vi "ReadUserExpressions.vi"(8 "error in (no error)":errorcluster, 11 "object in":refnum<class "execute_reply Message.lvclass">) -> (0 "error out":errorcluster, 2 "User Expressions":variant, 3 "object out":refnum<class "execute_reply Message.lvclass">)   [LabVIEW 2018, in "ClientMessaging.lvlib" / "execute_reply Message.lvclass"]
uses:
  execute_reply Message.lvclass
  execute_reply Message.lvclass/execute_reply Message.ctl
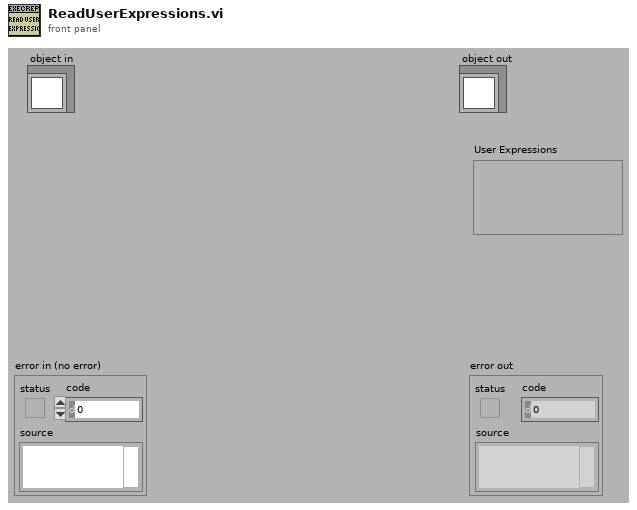
[diagram p1: front panel]
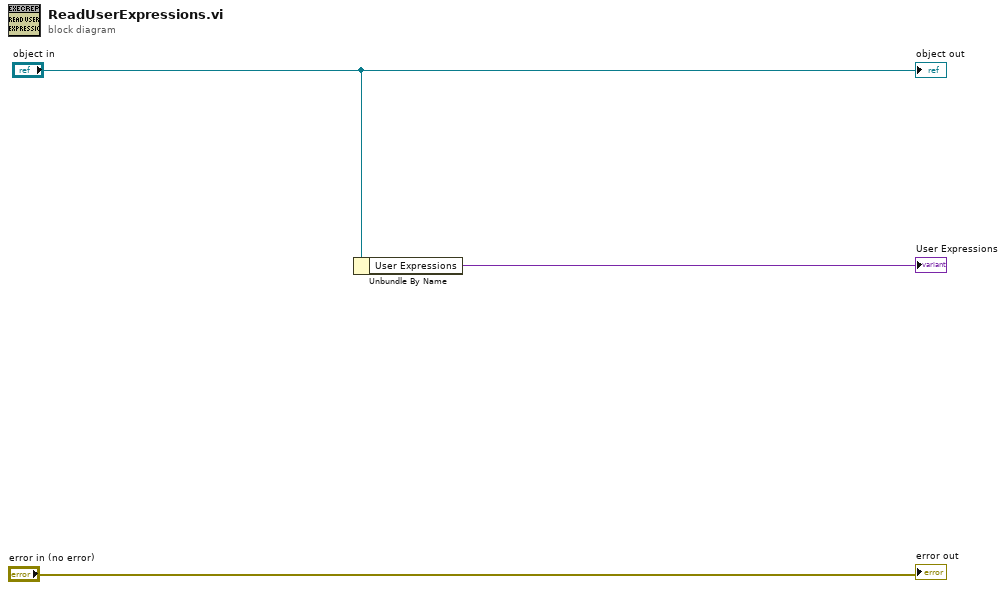
[diagram p0: block diagram]
diagram:
  n1 = Unbundle By Name("object in") -> ("User Expressions"=→"User Expressions":variant)
  "error out" <- "error in (no error)"
  "object out" <- "object in"
